vi "RT DI DAQ.vi"(11 "Queue ref":T1) -> ()   [LabVIEW 2022 SP3]
uses:
  RT Controls/RT All Queue.ctl
  RT Controls/RT DAQ case.ctl
  RT Controls/RT All Loop Status.ctl
  <vilib>/DAQmx/read.llb/DAQmx Read (Digital 1D Wfm NChan NSamp).vi
  RT Create Task/RT DI Create Task.vi
  <vilib>/DAQmx/configure/timing.llb/DAQmx Timing (Sample Clock).vi
  <vilib>/DAQmx/configure/trigger.llb/DAQmx Start Trigger (Time).vi
  RT Sub VI's/RT Global.vi
  <vilib>/DAQmx/miscellaneous.llb/DAQmx Fill In Error Info.vi
panel:
  out "error out":errorcluster
  # "TC channel list"
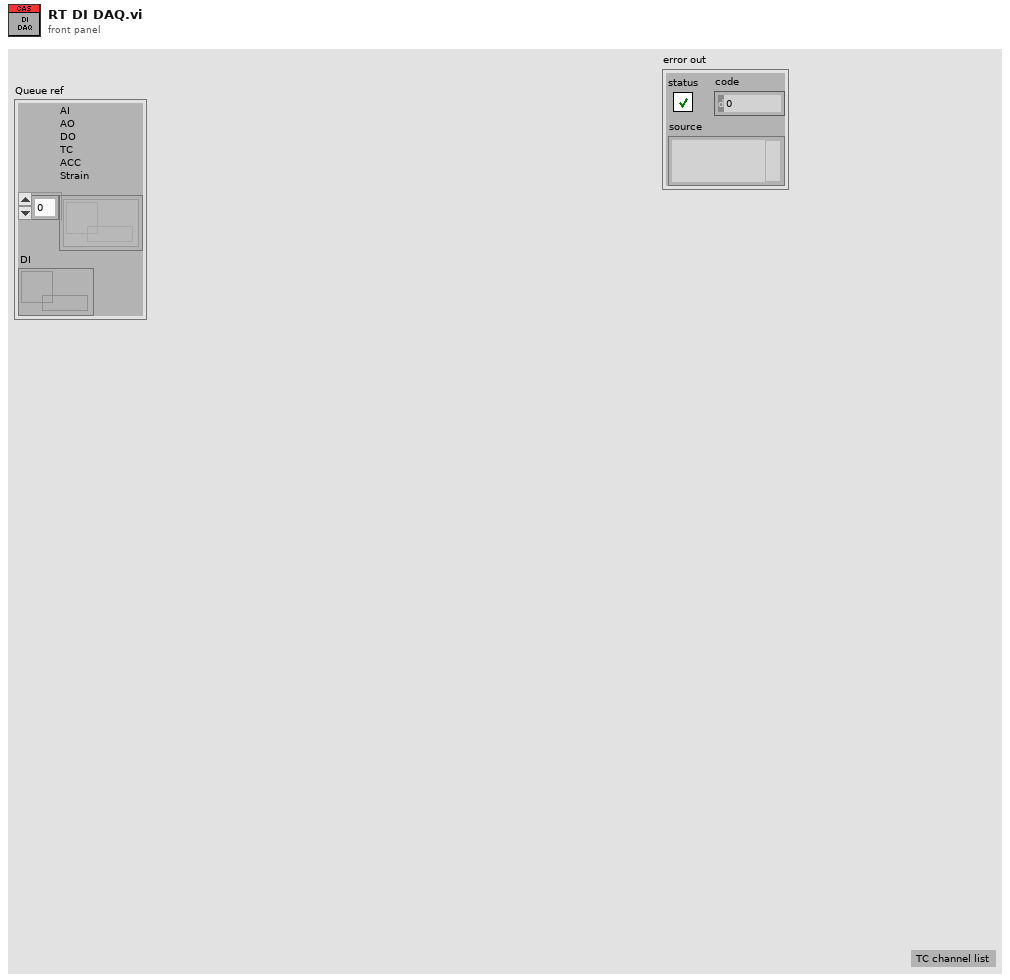
[diagram p1: front panel]
types:
  T1 = typedef "RT All Queue.ctl" = cluster{"AI\nAO\nDO\nTC\nACC\nStrain":refnum<queue>[], "DI":refnum<queue>}
  T2 = cluster{"in progress?":bool, "Start DAQ":refnum<notifier>, "task out":refnum<k21>, "DI":refnum<queue>, "SPC":i32}
  T3 = typedef "RT DAQ case.ctl" = enum16{"Initailise", "Create Task", "Polevent", "Acquire", "Stop DAQ", "Error", "Exit"}
  T4 = typedef "RT All Loop Status.ctl" = enum16{"AI", "AO", "DI", "DO", "TC", "Strain", "ACC", "RT", "Log", "Seq", "Sync"}
  T5 = enum16{"Init", "Read 'All'", "Read 'n'", "Read '1'", "Write '1'", "Write 'n'", "Write 'All'"}
  T6 = typedef "RT All Notifer.ctl" = cluster{"Start DAQ":refnum<notifier>, "Sequence":refnum<notifier>}
  T7 = cluster{"Analog input":bool, "Analog Output":bool, "Digital input":bool, "Digital output":bool, "Thermocouple":bool, "Strain Gauge":bool, "Accelerometer":bool}
  T8 = typedef "RT Config.ctl" = cluster{"AO config":cluster{"Channel_Name":string, "Channel_Number":string, "Default_Value":dbl, "Units":string}[], "AI config":cluster{"Channel_Name":string, "Channel_Number":string, "Pre_Scale_min":dbl, "Pre_Scale_max":dbl, "Sensor_min":dbl, "Sensor_max":dbl, "Units":string}[], "DI config":cluster{"Channel_Name":string, "Channel_Number":string, "Default_Value":bool, "Units":bool}[], "DO config":cluster{"Channel_Name":string, "Channel_Number":string, "Default_Value":bool, "Units":bool}[], "TC config":cluster{"Channel_Name":string, "Channel_Number":string, "Pre_Scale_min":dbl, "Pre_Scale_max":dbl, "units":i32, " type":i32}[], "ACC config":cluster{"Channel_Name":string, "Channel_Number":string, "Pre_Scale_min":dbl, "Pre_Scale_max":dbl, "Terminal configuration":i32, "Sensitivity":dbl, "Sensitivity units":i32}[], "SG config":cluster{"Channel_Name":string, "Channel_Number":string, "Pre_Scale_min":dbl, "Pre_Scale_max":dbl}[], "Strain Gauge Settings":cluster{"poisson ratio":dbl, "nominal gage resistance":dbl, "gage factor":dbl}, "Bridge Settings ":cluster{"strain configuration":i32, "lead wire resistance":dbl, "initial bridge voltage":dbl, "voltage excitation source":i32, "voltage excitation value":dbl}, "Sample Rate":cluster{"AI Sample Rate":dbl, "AO Sample Rate":dbl, "DI Sample Rate":dbl, "TC Sample Rate":dbl, "DO Sample Rate":dbl, "SG Sample Rate":dbl, "ACC Sample Rate":dbl}}
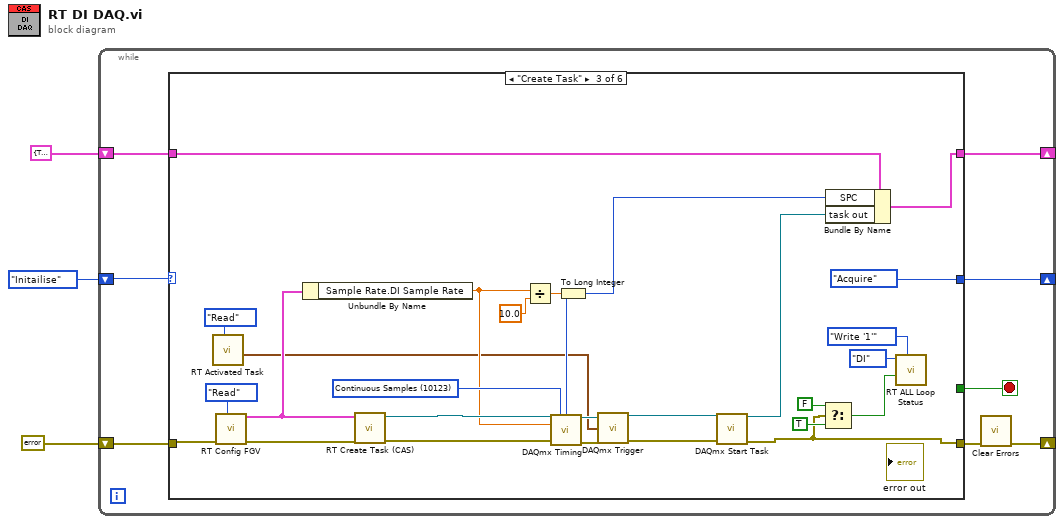
[diagram p0: block diagram]
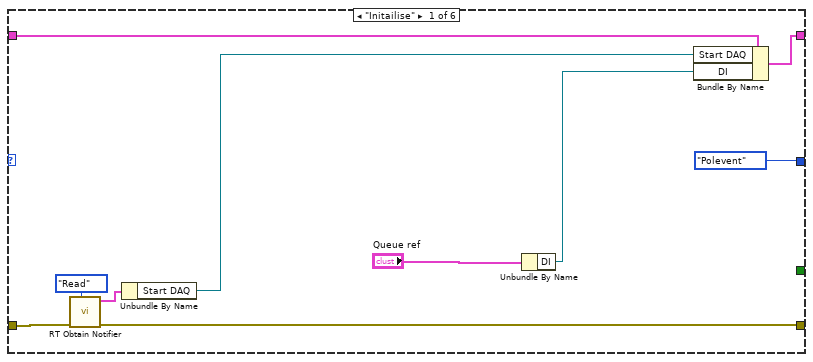
[diagram p2: hidden frame]
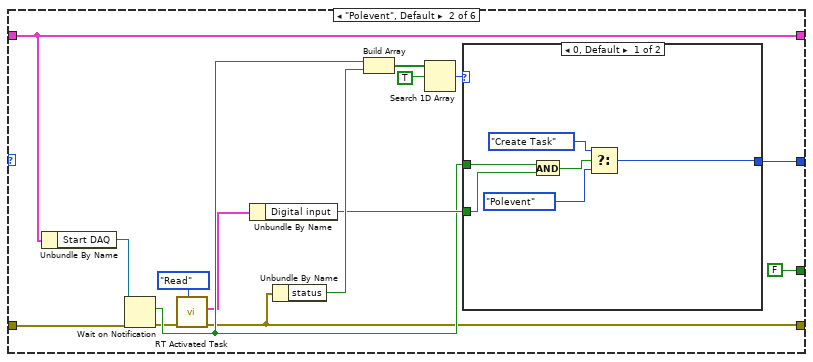
[diagram p3: hidden frame]
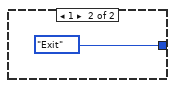
[diagram p4: hidden frame]
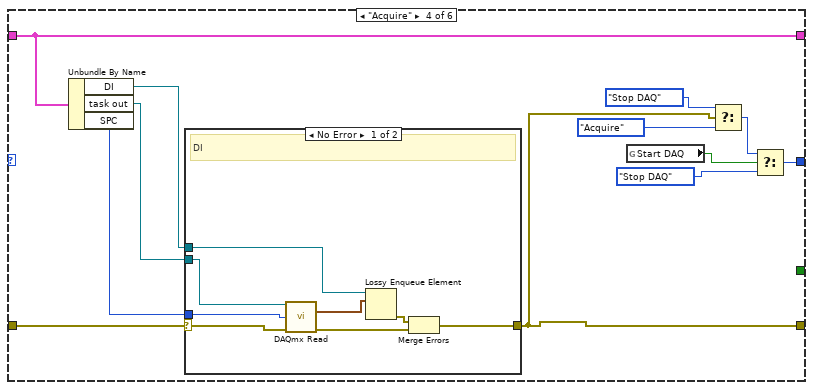
[diagram p5: hidden frame]
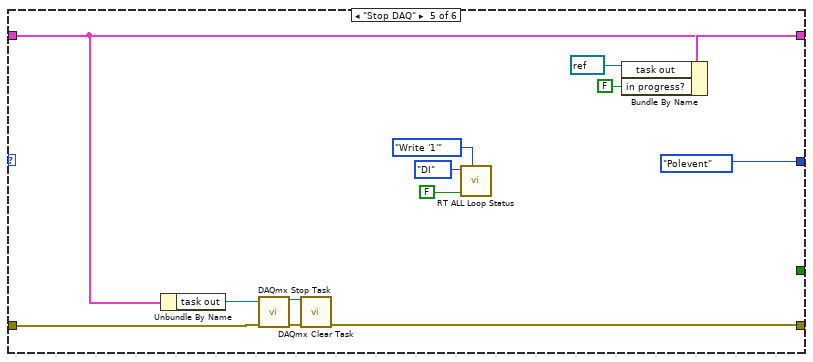
[diagram p7: hidden frame]
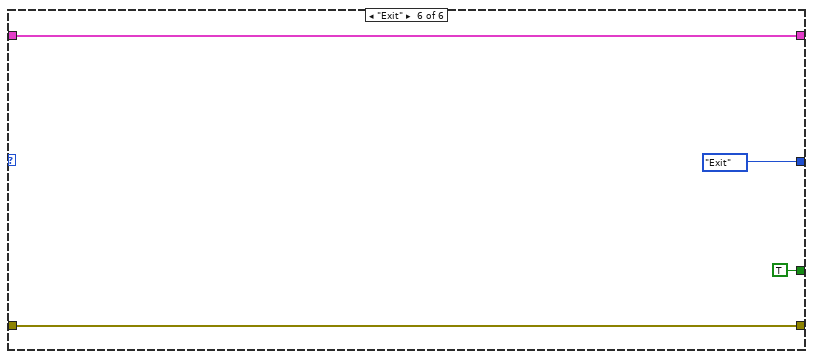
[diagram p8: hidden frame]
diagram:
  n1 = while {
    shift-right: [w4] -> _
    shift-left: errorcluster {"status"=FALSE, "code"=0, "source"=""} ("error out") -> [w10]
    shift-right: [w8] -> _
    shift-left: T2 {"in progress?"=TRUE, "Start DAQ"=refnum, "task out"="", "DI"=refnum, "SPC"=0} -> [w9]
    shift-right: [w7] -> _
    shift-left: RT_DAQ_case."Initailise" -> [w6]
    stop <- w11 stop-if-true
    n2 = case shown="\"Create Task\"" w6 {
      tunnel: [_ FALSE _ _ _ TRUE] -> w11
      tunnel: w10 -> [w15 w26 w62 w79 w98 w108]
      tunnel: [w14 w22 w65 w76 w99 w108] -> w5
      tunnel: w9 -> [w21 w34 w70 w80 w103 w107]
      tunnel: [w19 w34 w69 w80 w104 w107] -> w8
      tunnel: [RT_DAQ_case."Polevent" w35 RT_DAQ_case."Acquire" w81 RT_DAQ_case."Polevent" RT_DAQ_case."Exit"] -> w7
      frame "Initailise" {
        n3 = call "RT Obtain Notifier.vi"("Case"=enum16{"Obtain", "Read"}."Read", "error in (no error)"=w15) -> ("error out"=w14:errorcluster, "All Notifier"=w13:T6)  [unwired: 8 in]
        n4 = Unbundle By Name(w13) -> ("Start DAQ"=w20:refnum<notifier>)
        n5 = Unbundle By Name("Queue ref") -> ("DI"=w12:refnum<queue>)
        n6 = Bundle By Name(cluster=w21, "Start DAQ"=w20, "DI"=w12) -> (w19:T2)
      }
      frame "Polevent", Default {
        n7 = Unbundle By Name(w34) -> ("Start DAQ"=w33:refnum<notifier>)
        n8 = Wait on Notification(notifier=w33, error in (no error)=w26) -> (notification=w27:bool, error out=w23:errorcluster)  [unwired: 2 in, 2 out]
        n9 = call "RT Activated Task.vi"("Enum"=enum16{"Read", "Write"}."Read", "error in (no error)"=w23) -> ("error out"=w22:errorcluster, "Activate Task 2"=w25:T7)  [unwired: 7 in, 1 out]
        n10 = Unbundle By Name(w25) -> ("Digital input"=w28:bool)
        n11 = Unbundle By Name(w22) -> ("status"=w32:bool)
        n12 = Build Array(w27, w32) -> (w31:bool[])
        n13 = Search 1D Array(1D array=w31, element=TRUE) -> (index of element=w29:i32)  [unwired: 1 in]
        n14 = case shown="0, Default" w29 {
          tunnel: [w42 RT_DAQ_case."Exit"] -> w35
          tunnel: w28 -> [w40 _]
          tunnel: w27 -> [w39 _]
          frame 0, Default {
            n15 = And(x=w39, y=w40) -> (x .and. y?=w41:bool)
            n16 = Select(t=RT_DAQ_case."Create Task", s=w41, f=RT_DAQ_case."Polevent") -> (s? t:f=w42:T3)
          }
          frame 1 {
          }
        }
      }
      frame "Create Task" {
        w68 = 10123 items=["Finite Samples"=10178, "Continuous Samples"=10123, "Hardware Timed Single Point"=12522] ("sample mode")
        n17 = call "RT Activated Task.vi"("Enum"=enum16{"Read", "Write"}."Read") -> ("Start Time"=w45:timestamp)  [unwired: 8 in, 2 out]
        n18 = call "RT Config FGV.vi"("Enum"=enum16{"Read", "Write"}."Read", "error in (no error)"=w62) -> ("error out"=w61:errorcluster, "Data out"=w54:T8)  [unwired: 8 in]
        n19 = Unbundle By Name(w54) -> ("Sample Rate.DI Sample Rate"=w53:dbl)
        n20 = call-poly "RT Create Task (CAS).vi"("error in"=w61, "Config"=w54) -> ("error out"=w60:errorcluster, "DI Task"=w59:refnum<k21>)  [unwired: 7 in, 1 out]
        n21 = Divide(x=w53, y=10.0) -> (x/y=w51:dbl)
        n22 = To Long Integer(number=w51) -> (32bit integer=w50:i32)
        n23 = call-poly <vilib>:"DAQmx Timing.vi"("task/channels in"=w59, "sample mode"=w68, "samples per channel"=w50, "rate"=w53, "error in"=w60) -> ("task out"=w49:refnum<k21>, "error out"=w48:errorcluster)  [unwired: 9 in]
        n24 = call-poly <vilib>:"DAQmx Trigger.vi"("task/channels in"=w49, "when"=w45, "error in"=w48) -> ("task out"=w47:refnum<k21>, "error out"=w46:errorcluster)  [unwired: 11 in]
        n25 = call <vilib>:"DAQmx Start Task.vi"("task/channels in"=w47, "error in"=w46) -> ("task out"=w64:refnum<k21>, "error out"=w65:errorcluster)  [unwired: 12 in]
        n26 = Select(t=FALSE, s=w65, f=TRUE) -> (s? t:f=w56:bool)
        n27 = Bundle By Name(cluster=w70, "SPC"=w50, "task out"=w64) -> (w69:T2)
        n28 = call "RT ALL Loop Status.vi"("Option"=T5."Write '1'", "Status"=w56, "Loop"=RT_All_Loop_Status."DI") -> ()  [unwired: 6 in, 3 out]
      }
      frame "Acquire" {
        n29 = Unbundle By Name(w80) -> ("DI"=w78:refnum<queue>, "task out"=w77:refnum<k21>, "SPC"=w71:i32)
        n30 = case shown="No Error" w79 {
          selector: w79 -> [w87 w91]
          tunnel: w77 -> [w86 _]
          tunnel: [w88 w91] -> w76
          tunnel: w78 -> [w84 _]
          tunnel: w71 -> [w83 _]
          frame No Error {
            # "DI"
            n31 = call-poly <vilib>:"DAQmx Read.vi"("task/channels in"=w86, "number of samples per channel"=w83, "error in"=w87) -> ("data"=w85:digitalwaveform[], "error out"=w89:errorcluster)  [unwired: 10 in, 1 out]
            n32 = Lossy Enqueue Element(queue=w84, element=w85) -> (error out=w90:errorcluster)  [unwired: 1 in, 3 out]
            n33 = Merge Errors(w90, w89) -> (w88:errorcluster)
          }
          frame Error {
          }
        }
        n34 = global read "RT Global.vi" "Start DAQ"() -> (w72:bool)
        n35 = Select(t=RT_DAQ_case."Stop DAQ", s=w76, f=RT_DAQ_case."Acquire") -> (s? t:f=w82:T3)
        n36 = Select(t=w82, s=w72, f=RT_DAQ_case."Stop DAQ") -> (s? t:f=w81:T3)
      }
      frame "Stop DAQ" {
        n37 = Unbundle By Name(w103) -> ("task out"=w97:refnum<k21>)
        n38 = call <vilib>:"DAQmx Stop Task.vi"("task/channels in"=w97, "error in"=w98) -> ("task out"=w96:refnum<k21>, "error out"=w100:errorcluster)  [unwired: 12 in]
        n39 = call <vilib>:"DAQmx Clear Task.vi"("task in"=w96, "error in"=w100) -> ("error out"=w99:errorcluster)  [unwired: 13 in]
        n40 = call "RT ALL Loop Status.vi"("Option"=T5."Write '1'", "Status"=FALSE, "Loop"=RT_All_Loop_Status."DI") -> ()  [unwired: 6 in, 3 out]
        n41 = Bundle By Name(cluster=w103, "task out"=refnum<k21> refnum, "in progress?"=FALSE) -> (w104:T2)
      }
      frame "Exit" {
      }
    }
    n42 = call <vilib>:"Clear Errors.vi"("error in (no error)"=w5) -> ("error out"=w4:errorcluster)  [unwired: 5 in, 1 out]
  }
